vi "MAIN RT V2.vi"   [LabVIEW 2019]
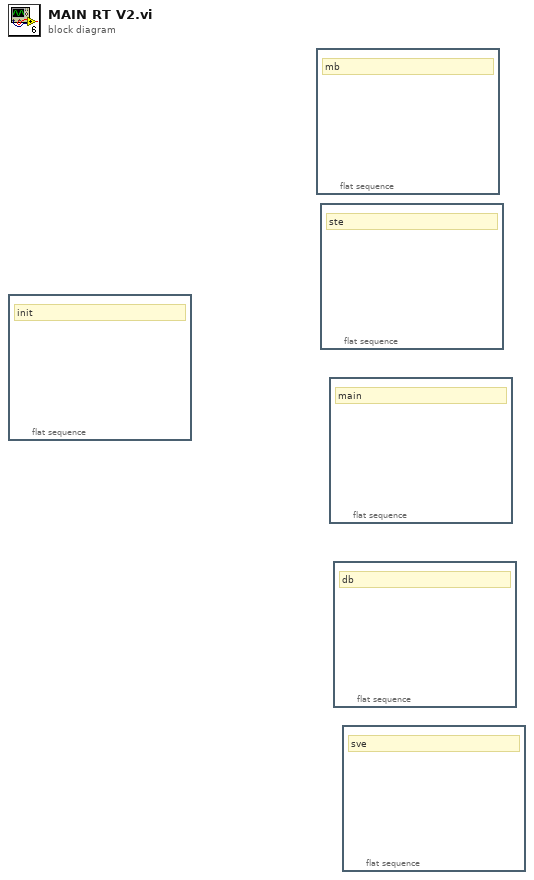
[diagram p0: block diagram]
diagram:
  n1 = flat-sequence {
    frame #0 {
      # "init"
    }
  }
  n2 = flat-sequence {
    frame #0 {
      # "mb"
    }
  }
  n3 = flat-sequence {
    frame #0 {
      # "ste"
    }
  }
  n4 = flat-sequence {
    frame #0 {
      # "main"
    }
  }
  n5 = flat-sequence {
    frame #0 {
      # "db"
    }
  }
  n6 = flat-sequence {
    frame #0 {
      # "sve"
    }
  }
